vi "DAQ_6001_ch1_test.vi"(2 "number of samples":i32=100, 3 "rate":dbl=1000.0) -> (0 "vol_out":dbl, 1 "data 2":dynamicdata(graph) caption="data")   [LabVIEW 2021]
panel:
  in  "stop":bool
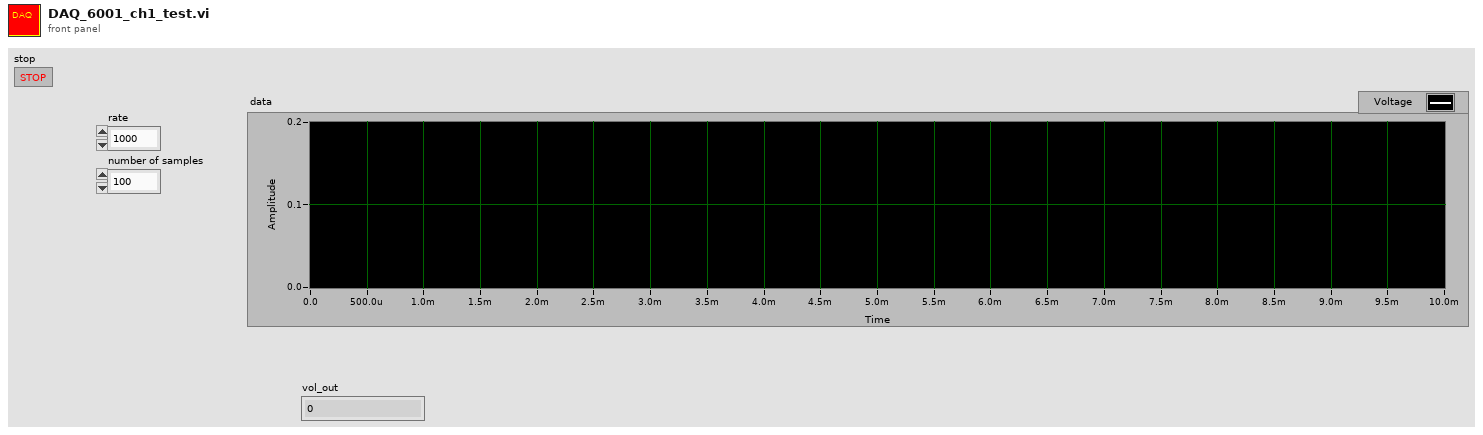
[diagram p1: front panel]
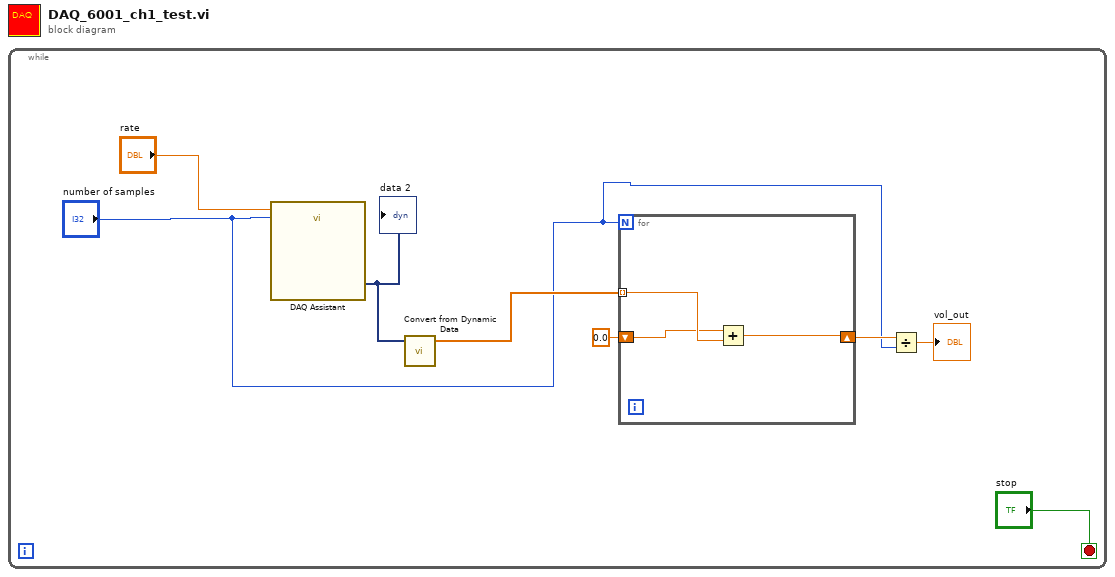
[diagram p0: block diagram]
diagram:
  n1 = while {
    stop <- "stop" stop-if-true
    n2 = call "DAQ Assistant"("rate"="rate", "number of samples"="number of samples") -> ("data"=w7:dynamicdata)  [unwired: 15 in, 2 out]
    "data 2" <- w7
    n3 = call "Convert from Dynamic Data"("Dynamic Data Type"=w7) -> ("Array"=w6:dbl[])  [unwired: 3 in]
    n4 = for {
      N: "number of samples" -> [_]
      tunnel: w6 -> [w11] mode=indexing
      shift-right: [w10] -> w4
      shift-left: 0.0 -> [w9]
      n5 = Add(x=w9, y=w11) -> (x+y=w10:dbl)
    }
    n6 = Divide(x=w4, y="number of samples") -> (x/y=→"vol_out":dbl)
  }
